vi "Create_Steps_List.vi"(0 "Steps List In":T1[](array[typedef])=[{"Wash States"=enum."Under Body Wash", "Expected Vehicle Pos"=1, "Step duration"=0}, {"Wash States"=enum."Bug Remover", "Expected Vehicle Pos"=1, "Step duration"=0}, {"Wash States"=enum."Pre-Soak", "Expected Vehicle Pos"=2, "Step duration"=0}, {"Wash States"=enum."High Pressure Wash", "Expected Vehicle Pos"=2, "Step duration"=0}, {"Wash States"=enum."Low Pressure Wax", "Expected Vehicle Pos"=2, "Step duration"=20}, {"Wash States"=enum."Spot Free Rinse", "Expected Vehicle Pos"=2, "Step duration"=0}, {"Wash States"=enum."Tire Shine Foam", "Expected Vehicle Pos"=3, "Step duration"=0}, {"Wash States"=enum."Air Dry", "Expected Vehicle Pos"=3, "Step duration"=50}], 1 "Buttons In":bool[](array[boolean])) -> (7 "Steps List Out":T1[](array[typedef]) {"Step duration" format="%<%H:%M:%S>t"})   [LabVIEW 2019]
uses:
  #typedef_WashStepInfo.ctl
  #typedef_WashStates.ctl
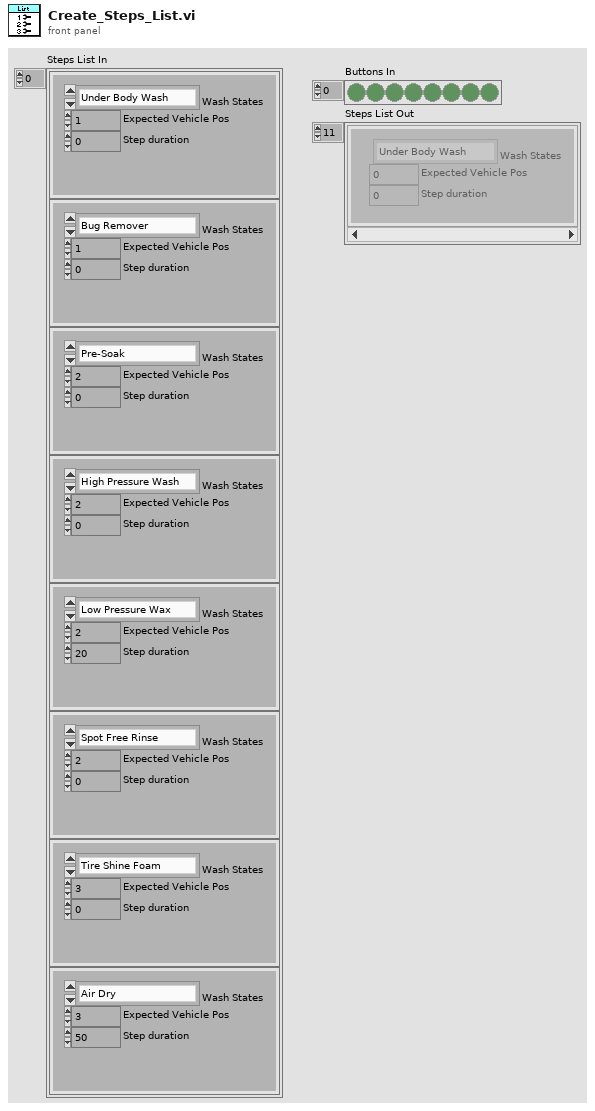
[diagram p1: front panel]
types:
  T1 = typedef "#typedef_WashStepInfo.ctl" = cluster{"Wash States":T2, "Expected Vehicle Pos":i32, "Step duration":i32}
  T2 = typedef "#typedef_WashStates.ctl" = enum16{"Under Body Wash", "Bug Remover", "Pre-Soak", "High Pressure Wash", "Low Pressure Wax", "Spot Free Rinse", "Tire Shine Foam", "Air Dry"}
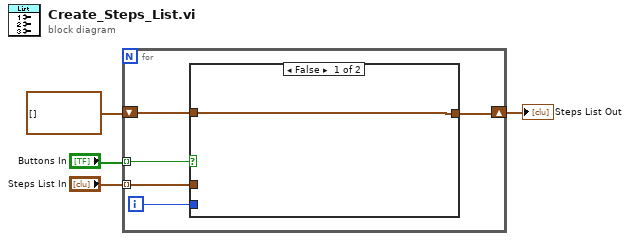
[diagram p0: block diagram]
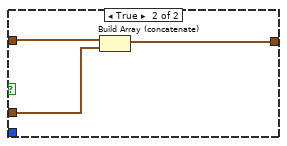
[diagram p2: hidden frame]
diagram:
  n1 = for {
    tunnel: "Buttons In" -> [w9] mode=indexing
    tunnel: "Steps List In" -> [w7] mode=indexing
    shift-right: [w5] -> w1
    shift-left: T1[] [] ("Steps List In") -> [w6]
    i -> [w8]
    n2 = case shown="False" w9 {
      tunnel: w8 -> [_ _]
      tunnel: w7 -> [_ w12]
      tunnel: w6 -> [w10 w13]
      tunnel: [w10 w11] -> w5
      frame False {
      }
      frame True {
        n3 = Build Array (concatenate)(w13, w12) -> (w11:T1[])
      }
    }
  }
  "Steps List Out" <- w1
